vi "executeCommand.vi"(8 "error in (no error)":errorcluster, 9 "parameter":variant, 10 "monoCommand":T2, 11 "MonoCommunicator in":refnum<class "MonoCommunicator.lvclass">) -> (0 "error out":errorcluster, 2 "answer":string, 3 "MonoCommunicator out":refnum<class "MonoCommunicator.lvclass">)   [LabVIEW 2016, in "MonoCommunicator.lvclass"]
uses:
  MonoCommunicator.lvclass
  Typedefs/MonoCommand.ctl
  Typedefs/GratingType.ctl
  Typedefs/SlitType.ctl
  Typedefs/wavelength.ctl
  MonoCommunicator.lvclass/MonoCommunicator.ctl
  Typedefs/AckType.ctl
  Typedefs/slitWidth.ctl
  Typedefs/slit.ctl
panel:
  in  "GratingType":T1=enum."Red"
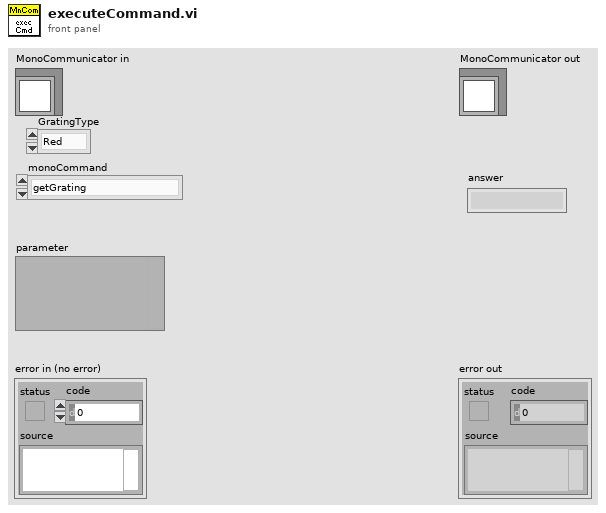
[diagram p1: front panel]
types:
  T1 = typedef "GratingType.ctl" = enum16{"Blue", "Red", "Mirror"}
  T2 = typedef "MonoCommand.ctl" = enum16{"getGrating", "getFrontEntranceSlitPosition", "getFrontExitSlitPosition", "getWavelength", "setWavelength", "setGrating", "setFrontEntranceSlitPosition", "setFrontExitSlitPosition", "calibrateWavelength", "getStatus", "Unknown", "reset"}
  T3 = typedef "SlitType.ctl" = enum16{"Front Entrance", "Side Entrance", "Front Exit", "Side Exit", "First Intermediate", "Second Intermediate"}
  T4 = typedef "wavelength.ctl" = dbl
  T5 = typedef "AckType.ctl" = enum16{"OK", "OutOfRange", "Unknown", "Busy", "Rejected"}
  T6 = typedef "slitWidth.ctl" = dbl
  T7 = typedef "slit.ctl" = cluster{"SlitType":T3, "Width":T6}
  T8 = typedef "Settings.lvlib/ConfigurationTypedefs.lvlib/MonochromatorSettings.ctl" = cluster{"Force Init":bool, "WavelengthMin":T4, "WavelengthMax":T4, "SlitWidthMin":T6, "SlitWidthMax":T6}
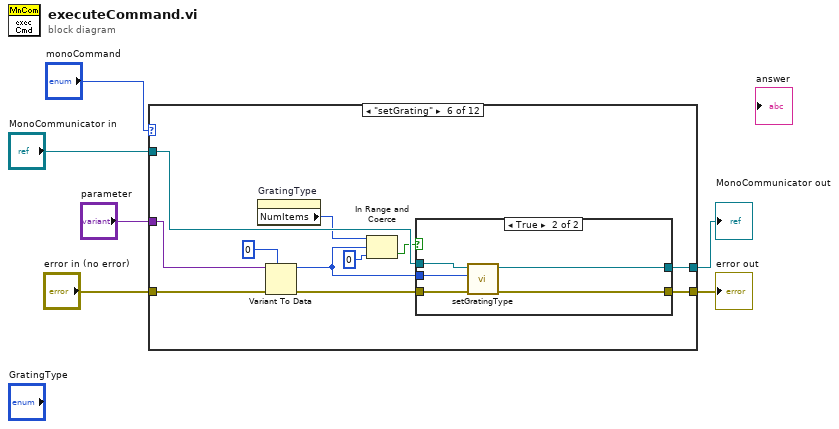
[diagram p0: block diagram]
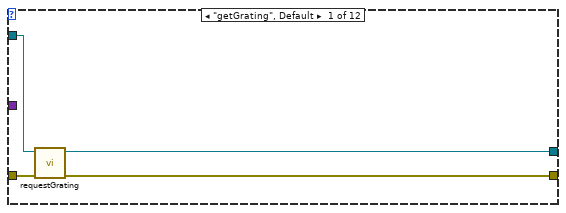
[diagram p2: hidden frame]
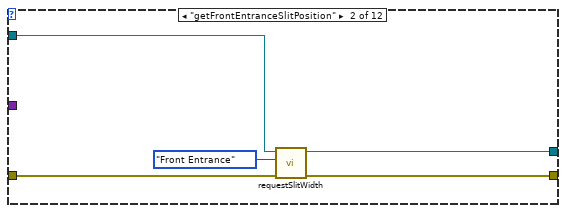
[diagram p3: hidden frame]
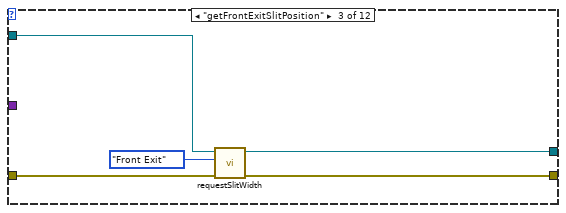
[diagram p4: hidden frame]
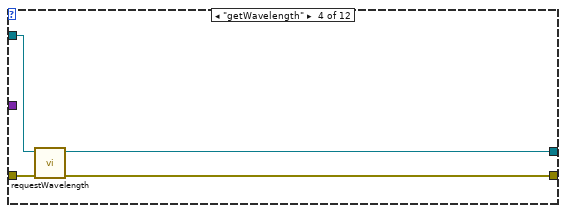
[diagram p5: hidden frame]
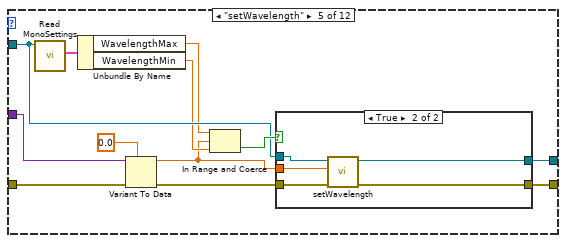
[diagram p6: hidden frame]
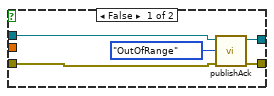
[diagram p7: hidden frame]
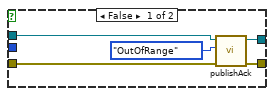
[diagram p8: hidden frame]
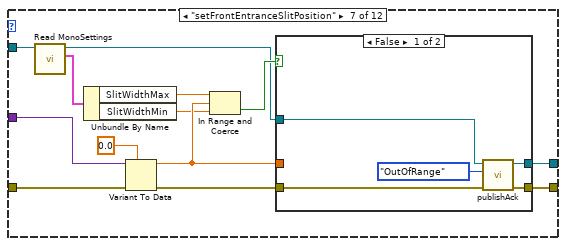
[diagram p9: hidden frame]
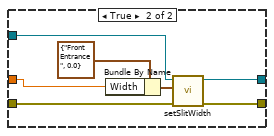
[diagram p10: hidden frame]
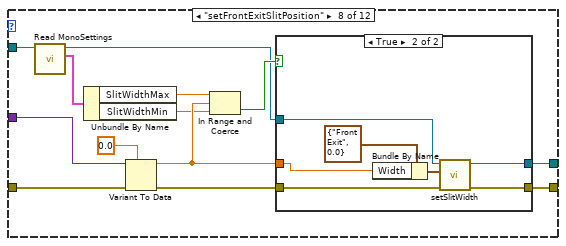
[diagram p11: hidden frame]
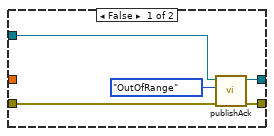
[diagram p12: hidden frame]
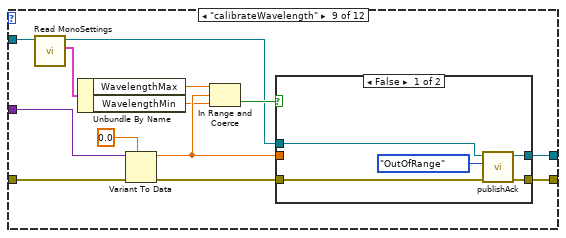
[diagram p13: hidden frame]
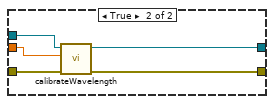
[diagram p14: hidden frame]
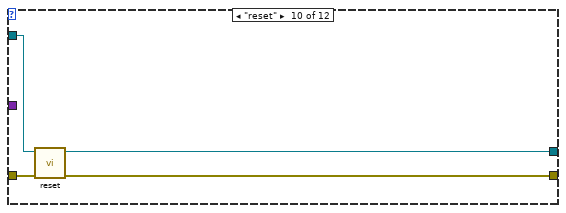
[diagram p15: hidden frame]
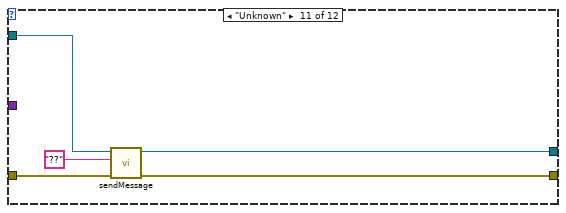
[diagram p16: hidden frame]
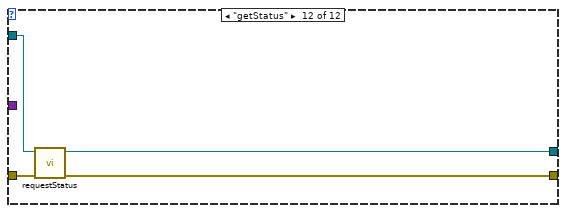
[diagram p17: hidden frame]
diagram:
  n1 = case shown="\"setGrating\"" "monoCommand" {
    tunnel: "MonoCommunicator in" -> [w7 w15 w20 w24 w28 w52 w72 w97 w122 w141 w149 w150]
    tunnel: [w8 w14 w19 w23 w36 w56 w79 w104 w130 w142 w148 w151] -> w4
    tunnel: "error in (no error)" -> [w10 w12 w17 w21 w34 w55 w75 w102 w128 w144 w147 w153]
    tunnel: [w9 w13 w18 w22 w35 w57 w80 w100 w129 w143 w146 w152] -> w2
    tunnel: "parameter" -> [_ _ _ _ w32 w53 w77 w103 w125 _ _ _]
    frame "getGrating", Default {
      n2 = call-dynamic "requestGrating.vi"("error in (no error)"=w10, "MonoCommunicator in"=w7) -> ("error out"=w9:errorcluster, "MonoCommunicator out"=w8:refnum<class "MonoCommunicator.lvclass">)  [unwired: 8 in]
    }
    frame "getFrontEntranceSlitPosition" {
      n3 = call-dynamic "requestSlitWidth.vi"("error in (no error)"=w12, "SlitType"=SlitType."Front Entrance", "MonoCommunicator in"=w15) -> ("error out"=w13:errorcluster, "MonoCommunicator out"=w14:refnum<class "MonoCommunicator.lvclass">)  [unwired: 7 in]
    }
    frame "getFrontExitSlitPosition" {
      n4 = call-dynamic "requestSlitWidth.vi"("error in (no error)"=w17, "SlitType"=SlitType."Front Exit", "MonoCommunicator in"=w20) -> ("error out"=w18:errorcluster, "MonoCommunicator out"=w19:refnum<class "MonoCommunicator.lvclass">)  [unwired: 7 in]
    }
    frame "getWavelength" {
      n5 = call-dynamic "requestWavelength.vi"("error in (no error)"=w21, "MonoCommunicator in"=w24) -> ("error out"=w22:errorcluster, "MonoCommunicator out"=w23:refnum<class "MonoCommunicator.lvclass">)  [unwired: 8 in]
    }
    frame "setWavelength" {
      n6 = call "Read MonoSettings.vi"("MonoCommunicator in"=w28) -> ("MonoSettings"=w29:T8)  [unwired: 8 in, 2 out]
      n7 = Unbundle By Name(w29) -> ("WavelengthMax"=w27:T4, "WavelengthMin"=w26:T4)
      n8 = Variant To Data(error in=w34, type=T4 0.0 ("wavelength"), Variant=w32) -> (data=w25:T4, error out=w33:errorcluster)
      n9 = In Range and Coerce(upper limit=w27, x=w25, lower limit=w26) -> (In Range?=w30:bool)  [unwired: 1 out]
      n10 = case shown="True" w30 {
        tunnel: w28 -> [w39 w46]
        tunnel: [w38 w45] -> w36
        tunnel: [w37 w44] -> w35
        tunnel: w33 -> [w40 w43]
        tunnel: w25 -> [_ w42]
        frame False {
          n11 = call "publishAck.vi"("error in (no error)"=w40, "AckType"=AckType."OutOfRange", "MonoCommunicator in"=w39) -> ("error out"=w37:errorcluster, "MonoCommunicator out"=w38:refnum<class "MonoCommunicator.lvclass">)  [unwired: 7 in]
        }
        frame True {
          n12 = call-dynamic "setWavelength.vi"("error in (no error)"=w43, "wavelength"=w42, "MonoCommunicator in"=w46) -> ("error out"=w44:errorcluster, "MonoCommunicator out"=w45:refnum<class "MonoCommunicator.lvclass">)  [unwired: 7 in]
        }
      }
    }
    frame "setGrating" {
      n13 = property on="GratingType" class="Enum (strict)"() -> ("NumItems"=w47:u32)  [unwired: 2 in, 2 out]
      n14 = Variant To Data(error in=w55, type=u16 0, Variant=w53) -> (data=w49:u16, error out=w54:errorcluster)
      n15 = In Range and Coerce(upper limit=w47, x=w49, lower limit=u32 0) -> (In Range?=w48:bool)  [unwired: 1 out]
      n16 = case shown="True" w48 {
        tunnel: [w60 w67] -> w57
        tunnel: [w59 w66] -> w56
        tunnel: w54 -> [w61 w65]
        tunnel: w49 -> [_ w64]
        tunnel: w52 -> [w58 w63]
        frame False {
          n17 = call "publishAck.vi"("error in (no error)"=w61, "AckType"=AckType."OutOfRange", "MonoCommunicator in"=w58) -> ("error out"=w60:errorcluster, "MonoCommunicator out"=w59:refnum<class "MonoCommunicator.lvclass">)  [unwired: 7 in]
        }
        frame True {
          n18 = call-dynamic "setGratingType.vi"("error in (no error)"=w65, "GratingType"=w64, "MonoCommunicator in"=w63) -> ("error out"=w67:errorcluster, "MonoCommunicator out"=w66:refnum<class "MonoCommunicator.lvclass">)  [unwired: 7 in]
        }
      }
    }
    frame "setFrontEntranceSlitPosition" {
      n19 = call "Read MonoSettings.vi"("MonoCommunicator in"=w72) -> ("MonoSettings"=w70:T8, "MonoCommunicator out"=w71:refnum<class "MonoCommunicator.lvclass">)  [unwired: 8 in, 1 out]
      n20 = Unbundle By Name(w70) -> ("SlitWidthMax"=w68:T6, "SlitWidthMin"=w69:T6)
      n21 = Variant To Data(error in=w75, type=T6 0.0 ("position"), Variant=w77) -> (data=w73:T6, error out=w76:errorcluster)
      n22 = In Range and Coerce(upper limit=w68, x=w73, lower limit=w69) -> (In Range?=w74:bool)  [unwired: 1 out]
      n23 = case shown="False" w74 {
        tunnel: [w84 w92] -> w80
        tunnel: [w83 w91] -> w79
        tunnel: w71 -> [w82 w90]
        tunnel: w76 -> [w85 w87]
        tunnel: w73 -> [_ w86]
        frame False {
          n24 = call "publishAck.vi"("error in (no error)"=w85, "AckType"=AckType."OutOfRange", "MonoCommunicator in"=w82) -> ("error out"=w84:errorcluster, "MonoCommunicator out"=w83:refnum<class "MonoCommunicator.lvclass">)  [unwired: 7 in]
        }
        frame True {
          n25 = Bundle By Name(cluster=T7 {"SlitType"=enum."Front Entrance", "Width"=0.0} ("position"), "Width"=w86) -> (w88:T7)
          n26 = call-dynamic "setSlitWidth.vi"("error in (no error)"=w87, "position"=w88, "MonoCommunicator in"=w90) -> ("error out"=w92:errorcluster, "MonoCommunicator out"=w91:refnum<class "MonoCommunicator.lvclass">)  [unwired: 7 in]
        }
      }
    }
    frame "setFrontExitSlitPosition" {
      n27 = call "Read MonoSettings.vi"("MonoCommunicator in"=w97) -> ("MonoSettings"=w95:T8, "MonoCommunicator out"=w96:refnum<class "MonoCommunicator.lvclass">)  [unwired: 8 in, 1 out]
      n28 = Unbundle By Name(w95) -> ("SlitWidthMax"=w93:T6, "SlitWidthMin"=w94:T6)
      n29 = Variant To Data(error in=w102, type=T6 0.0 ("position"), Variant=w103) -> (data=w99:T6, error out=w101:errorcluster)
      n30 = In Range and Coerce(upper limit=w93, x=w99, lower limit=w94) -> (In Range?=w98:bool)  [unwired: 1 out]
      n31 = case shown="True" w98 {
        tunnel: w99 -> [_ w115]
        tunnel: [w107 w114] -> w104
        tunnel: w96 -> [w108 w113]
        tunnel: w101 -> [w109 w112]
        tunnel: [w106 w111] -> w100
        frame False {
          n32 = call "publishAck.vi"("error in (no error)"=w109, "AckType"=AckType."OutOfRange", "MonoCommunicator in"=w108) -> ("error out"=w106:errorcluster, "MonoCommunicator out"=w107:refnum<class "MonoCommunicator.lvclass">)  [unwired: 7 in]
        }
        frame True {
          n33 = Bundle By Name(cluster=T7 {"SlitType"=enum."Front Exit", "Width"=0.0} ("position"), "Width"=w115) -> (w116:T7)
          n34 = call-dynamic "setSlitWidth.vi"("error in (no error)"=w112, "position"=w116, "MonoCommunicator in"=w113) -> ("error out"=w111:errorcluster, "MonoCommunicator out"=w114:refnum<class "MonoCommunicator.lvclass">)  [unwired: 7 in]
        }
      }
    }
    frame "calibrateWavelength" {
      n35 = call "Read MonoSettings.vi"("MonoCommunicator in"=w122) -> ("MonoSettings"=w120:T8, "MonoCommunicator out"=w121:refnum<class "MonoCommunicator.lvclass">)  [unwired: 8 in, 1 out]
      n36 = Unbundle By Name(w120) -> ("WavelengthMax"=w119:T4, "WavelengthMin"=w118:T4)
      n37 = Variant To Data(error in=w128, type=T4 0.0 ("wavelength"), Variant=w125) -> (data=w123:T4, error out=w127:errorcluster)
      n38 = In Range and Coerce(upper limit=w119, x=w123, lower limit=w118) -> (In Range?=w124:bool)  [unwired: 1 out]
      n39 = case shown="False" w124 {
        tunnel: w121 -> [w133 w140]
        tunnel: [w132 w139] -> w130
        tunnel: [w131 w138] -> w129
        tunnel: w127 -> [w134 w137]
        tunnel: w123 -> [_ w136]
        frame False {
          n40 = call "publishAck.vi"("error in (no error)"=w134, "AckType"=AckType."OutOfRange", "MonoCommunicator in"=w133) -> ("error out"=w131:errorcluster, "MonoCommunicator out"=w132:refnum<class "MonoCommunicator.lvclass">)  [unwired: 7 in]
        }
        frame True {
          n41 = call-dynamic "calibrateWavelength.vi"("error in (no error)"=w137, "wavelength"=w136, "MonoCommunicator in"=w140) -> ("error out"=w138:errorcluster, "MonoCommunicator out"=w139:refnum<class "MonoCommunicator.lvclass">)  [unwired: 7 in]
        }
      }
    }
    frame "reset" {
      n42 = call-dynamic "reset.vi"("error in (no error)"=w144, "MonoCommunicator in"=w141) -> ("error out"=w143:errorcluster, "MonoCommunicator out"=w142:refnum<class "MonoCommunicator.lvclass">)  [unwired: 8 in]
    }
    frame "Unknown" {
      n43 = call-dynamic "sendMessage.vi"("error in (no error)"=w147, "message"="??", "MonoCommunicator in"=w149) -> ("error out"=w146:errorcluster, "MonoCommunicator out"=w148:refnum<class "MonoCommunicator.lvclass">)  [unwired: 7 in]
    }
    frame "getStatus" {
      n44 = call-dynamic "requestStatus.vi"("error in (no error)"=w153, "MonoCommunicator in"=w150) -> ("error out"=w152:errorcluster, "MonoCommunicator out"=w151:refnum<class "MonoCommunicator.lvclass">)  [unwired: 8 in]
    }
  }
  "error out" <- w2
  "MonoCommunicator out" <- w4
